vi "Extract Newtwork Variable.vi"(8 "Saving":bool[](array[boolean]), 9 "Current":dbl[](array[numeric]), 10 "Array in":i32[](array[numeric]), 11 "Array 3":T1[](array[typedef]) {"Unit Type" items=["", "Viper", "Hawk", "Other"]; "Current" format="%.2f"; "Day Cycle Count" format="%04d"}) -> (3 "Array out":T1[](array[typedef]) {"Unit Type" items=["", "Viper", "Hawk", "Other"]; "Current" format="%.2f"; "Day Cycle Count" format="%04d"})   [LabVIEW 2012]
uses:
  Nufi/Newfi LDN/Washer.ctl
  Nufi/Newfi LDN/Washer Details.ctl
  Nufi/Newfi LDN/Unit Type.ctl
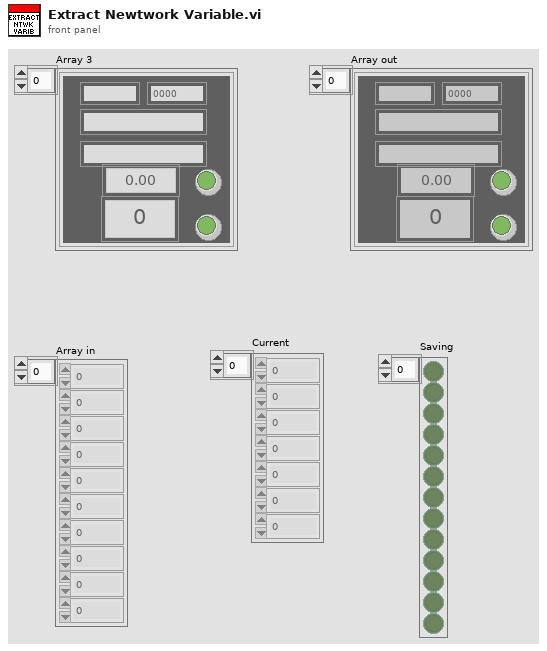
[diagram p1: front panel]
types:
  T1 = typedef "Washer.ctl" = cluster{"Serial Number":string, "Day Cycle Count":i32, "Station Label":string, "Status Color":u32, "Current Run Start Time":dbl, "Audit Alert":bool, "Washer Details":T2, "Board ID":string, "Boolean":bool, "RPM":u32, "Current":dbl, "Current Path":path, "Saving":bool, "Unit Type":T3}
  T2 = typedef "Washer Details.ctl" = cluster{"Cycle Count":string, "Status":string, "Notes":string, "Lab ID":string, "Total Time On":string, "TR Number":string}
  T3 = typedef "Unit Type.ctl" = u32
  T4 = cluster{"Serial Number":string, "Day Cycle Count":i32, "Station Label":string, "Status Color":u32, "Current Run Start Time":dbl, "Audit Alert":bool, "Washer Details":cluster{"Cycle Count":string, "Status":string, "Notes":string, "Lab ID":string, "Total Time On":string, "TR Number":string}, "Board ID":string, "Boolean":bool, "RPM":u32, "Current":dbl, "Current Path":path, "Saving":bool, "Unit Type":u32}
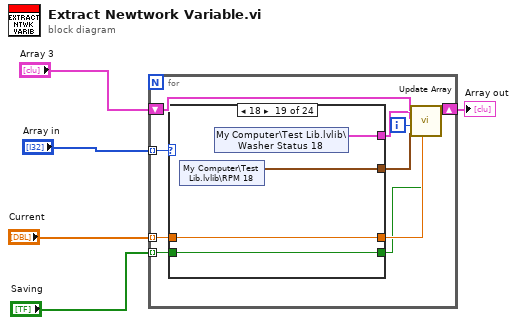
[diagram p0: block diagram]
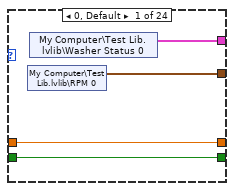
[diagram p2: hidden frame]
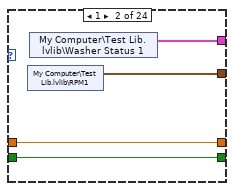
[diagram p3: hidden frame]
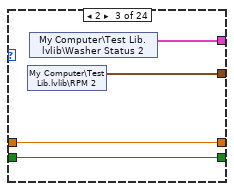
[diagram p4: hidden frame]
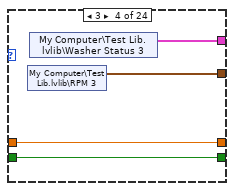
[diagram p5: hidden frame]
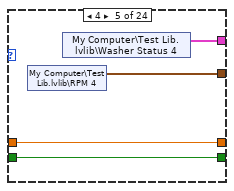
[diagram p6: hidden frame]
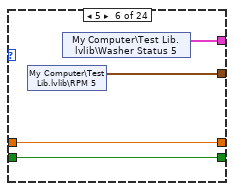
[diagram p7: hidden frame]
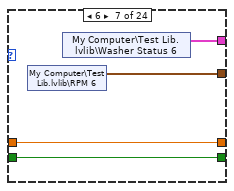
[diagram p8: hidden frame]
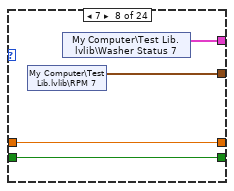
[diagram p9: hidden frame]
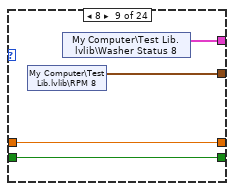
[diagram p10: hidden frame]
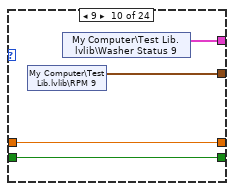
[diagram p11: hidden frame]
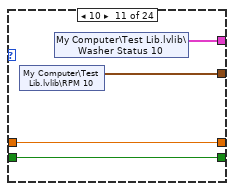
[diagram p12: hidden frame]
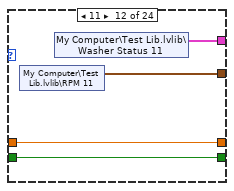
[diagram p13: hidden frame]
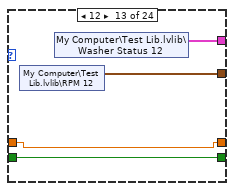
[diagram p14: hidden frame]
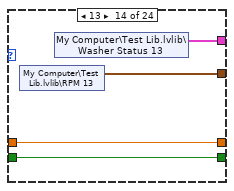
[diagram p15: hidden frame]
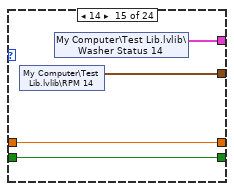
[diagram p16: hidden frame]
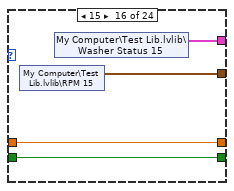
[diagram p17: hidden frame]
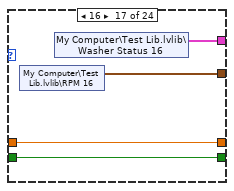
[diagram p18: hidden frame]
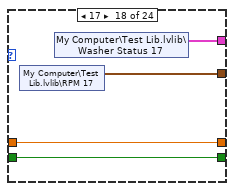
[diagram p19: hidden frame]
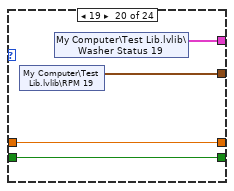
[diagram p20: hidden frame]
diagram:
  n1 = for {
    shift-right: [w14] -> w4
    shift-left: "Array 3" -> [w15]
    tunnel: "Array in" -> [w12] mode=indexing
    tunnel: "Current" -> [w9] mode=indexing
    tunnel: "Saving" -> [w7] mode=indexing
    i -> [w11]
    n2 = case shown="18" w12 {
      tunnel: [w19 w23 w27 w31 w35 w39 w43 w47 w51 w55 w59 w63 w67 w71 w75 w79 w83 w87 w91 w95 w99 w103 w107 w111] -> w13
      tunnel: [w18 w22 w26 w30 w34 w38 w42 w46 w50 w54 w58 w62 w66 w70 w74 w78 w82 w86 w90 w94 w98 w102 w106 w110] -> w10
      tunnel: [w17 w21 w25 w29 w33 w37 w41 w45 w49 w53 w57 w61 w65 w69 w73 w77 w81 w85 w89 w93 w97 w101 w105 w109] -> w8
      tunnel: w9 -> [w17 w21 w25 w29 w33 w37 w41 w45 w49 w53 w57 w61 w65 w69 w73 w77 w81 w85 w89 w93 w97 w101 w105 w109]
      tunnel: w7 -> [w16 w20 w24 w28 w32 w36 w40 w44 w48 w52 w56 w60 w64 w68 w72 w76 w80 w84 w88 w92 w96 w100 w104 w108]
      tunnel: [w16 w20 w24 w28 w32 w36 w40 w44 w48 w52 w56 w60 w64 w68 w72 w76 w80 w84 w88 w92 w96 w100 w104 w108] -> w6
      frame 0, Default {
        n3 = shared-variable "My Computer\\Test Lib.lvlib\\RPM 0"() -> (w18:cluster{"RPM":u32})  [unwired: 1 in, 1 out]
        n4 = shared-variable "My Computer\\Test Lib.lvlib\\Washer Status 0"() -> (w19:T4)  [unwired: 1 in, 1 out]
      }
      frame 1 {
        n5 = shared-variable "My Computer\\Test Lib.lvlib\\RPM1"() -> (w22:cluster{"RPM":u32})  [unwired: 1 in, 1 out]
        n6 = shared-variable "My Computer\\Test Lib.lvlib\\Washer Status 1"() -> (w23:T4)  [unwired: 1 in, 1 out]
      }
      frame 2 {
        n7 = shared-variable "My Computer\\Test Lib.lvlib\\RPM 2"() -> (w26:cluster{"RPM":u32})  [unwired: 1 in, 1 out]
        n8 = shared-variable "My Computer\\Test Lib.lvlib\\Washer Status 2"() -> (w27:T4)  [unwired: 1 in, 1 out]
      }
      frame 3 {
        n9 = shared-variable "My Computer\\Test Lib.lvlib\\RPM 3"() -> (w30:cluster{"RPM":u32})  [unwired: 1 in, 1 out]
        n10 = shared-variable "My Computer\\Test Lib.lvlib\\Washer Status 3"() -> (w31:T4)  [unwired: 1 in, 1 out]
      }
      frame 4 {
        n11 = shared-variable "My Computer\\Test Lib.lvlib\\RPM 4"() -> (w34:cluster{"RPM":u32})  [unwired: 1 in, 1 out]
        n12 = shared-variable "My Computer\\Test Lib.lvlib\\Washer Status 4"() -> (w35:T4)  [unwired: 1 in, 1 out]
      }
      frame 5 {
        n13 = shared-variable "My Computer\\Test Lib.lvlib\\RPM 5"() -> (w38:cluster{"RPM":u32})  [unwired: 1 in, 1 out]
        n14 = shared-variable "My Computer\\Test Lib.lvlib\\Washer Status 5"() -> (w39:T4)  [unwired: 1 in, 1 out]
      }
      frame 6 {
        n15 = shared-variable "My Computer\\Test Lib.lvlib\\RPM 6"() -> (w42:cluster{"RPM":u32})  [unwired: 1 in, 1 out]
        n16 = shared-variable "My Computer\\Test Lib.lvlib\\Washer Status 6"() -> (w43:T4)  [unwired: 1 in, 1 out]
      }
      frame 7 {
        n17 = shared-variable "My Computer\\Test Lib.lvlib\\RPM 7"() -> (w46:cluster{"RPM":u32})  [unwired: 1 in, 1 out]
        n18 = shared-variable "My Computer\\Test Lib.lvlib\\Washer Status 7"() -> (w47:T4)  [unwired: 1 in, 1 out]
      }
      frame 8 {
        n19 = shared-variable "My Computer\\Test Lib.lvlib\\RPM 8"() -> (w50:cluster{"RPM":u32})  [unwired: 1 in, 1 out]
        n20 = shared-variable "My Computer\\Test Lib.lvlib\\Washer Status 8"() -> (w51:T4)  [unwired: 1 in, 1 out]
      }
      frame 9 {
        n21 = shared-variable "My Computer\\Test Lib.lvlib\\RPM 9"() -> (w54:cluster{"RPM":u32})  [unwired: 1 in, 1 out]
        n22 = shared-variable "My Computer\\Test Lib.lvlib\\Washer Status 9"() -> (w55:T4)  [unwired: 1 in, 1 out]
      }
      frame 10 {
        n23 = shared-variable "My Computer\\Test Lib.lvlib\\RPM 10"() -> (w58:cluster{"RPM":u32})  [unwired: 1 in, 1 out]
        n24 = shared-variable "My Computer\\Test Lib.lvlib\\Washer Status 10"() -> (w59:T4)  [unwired: 1 in, 1 out]
      }
      frame 11 {
        n25 = shared-variable "My Computer\\Test Lib.lvlib\\RPM 11"() -> (w62:cluster{"RPM":u32})  [unwired: 1 in, 1 out]
        n26 = shared-variable "My Computer\\Test Lib.lvlib\\Washer Status 11"() -> (w63:T4)  [unwired: 1 in, 1 out]
      }
      frame 12 {
        n27 = shared-variable "My Computer\\Test Lib.lvlib\\RPM 12"() -> (w66:cluster{"RPM":u32})  [unwired: 1 in, 1 out]
        n28 = shared-variable "My Computer\\Test Lib.lvlib\\Washer Status 12"() -> (w67:T4)  [unwired: 1 in, 1 out]
      }
      frame 13 {
        n29 = shared-variable "My Computer\\Test Lib.lvlib\\RPM 13"() -> (w70:cluster{"RPM":u32})  [unwired: 1 in, 1 out]
        n30 = shared-variable "My Computer\\Test Lib.lvlib\\Washer Status 13"() -> (w71:T4)  [unwired: 1 in, 1 out]
      }
      frame 14 {
        n31 = shared-variable "My Computer\\Test Lib.lvlib\\RPM 14"() -> (w74:cluster{"RPM":u32})  [unwired: 1 in, 1 out]
        n32 = shared-variable "My Computer\\Test Lib.lvlib\\Washer Status 14"() -> (w75:T4)  [unwired: 1 in, 1 out]
      }
      frame 15 {
        n33 = shared-variable "My Computer\\Test Lib.lvlib\\RPM 15"() -> (w78:cluster{"RPM":u32})  [unwired: 1 in, 1 out]
        n34 = shared-variable "My Computer\\Test Lib.lvlib\\Washer Status 15"() -> (w79:T4)  [unwired: 1 in, 1 out]
      }
      frame 16 {
        n35 = shared-variable "My Computer\\Test Lib.lvlib\\RPM 16"() -> (w82:cluster{"RPM":u32})  [unwired: 1 in, 1 out]
        n36 = shared-variable "My Computer\\Test Lib.lvlib\\Washer Status 16"() -> (w83:T4)  [unwired: 1 in, 1 out]
      }
      frame 17 {
        n37 = shared-variable "My Computer\\Test Lib.lvlib\\RPM 17"() -> (w86:cluster{"RPM":u32})  [unwired: 1 in, 1 out]
        n38 = shared-variable "My Computer\\Test Lib.lvlib\\Washer Status 17"() -> (w87:T4)  [unwired: 1 in, 1 out]
      }
      frame 18 {
        n39 = shared-variable "My Computer\\Test Lib.lvlib\\RPM 18"() -> (w90:cluster{"RPM":u32})  [unwired: 1 in, 1 out]
        n40 = shared-variable "My Computer\\Test Lib.lvlib\\Washer Status 18"() -> (w91:T4)  [unwired: 1 in, 1 out]
      }
      frame 19 {
        n41 = shared-variable "My Computer\\Test Lib.lvlib\\RPM 19"() -> (w94:cluster{"RPM":u32})  [unwired: 1 in, 1 out]
        n42 = shared-variable "My Computer\\Test Lib.lvlib\\Washer Status 19"() -> (w95:T4)  [unwired: 1 in, 1 out]
      }
      frame 20 {
        n43 = shared-variable "My Computer\\Test Lib.lvlib\\RPM 20"() -> (w98:cluster{"RPM":u32})  [unwired: 1 in, 1 out]
        n44 = shared-variable "My Computer\\Test Lib.lvlib\\Washer Status 20"() -> (w99:T4)  [unwired: 1 in, 1 out]
      }
      frame 21 {
        n45 = shared-variable "My Computer\\Test Lib.lvlib\\RPM 21"() -> (w102:cluster{"RPM":u32})  [unwired: 1 in, 1 out]
        n46 = shared-variable "My Computer\\Test Lib.lvlib\\Washer Status 21"() -> (w103:T4)  [unwired: 1 in, 1 out]
      }
      frame 22 {
        n47 = shared-variable "My Computer\\Test Lib.lvlib\\RPM 22"() -> (w106:cluster{"RPM":u32})  [unwired: 1 in, 1 out]
        n48 = shared-variable "My Computer\\Test Lib.lvlib\\Washer Status 22"() -> (w107:T4)  [unwired: 1 in, 1 out]
      }
      frame 23 {
        n49 = shared-variable "My Computer\\Test Lib.lvlib\\RPM 23"() -> (w110:cluster{"RPM":u32})  [unwired: 1 in, 1 out]
        n50 = shared-variable "My Computer\\Test Lib.lvlib\\Washer Status 23"() -> (w111:T4)  [unwired: 1 in, 1 out]
      }
    }
    n51 = call "Update Array.vi"("Saving"=w6, "Current"=w8, "RPM and Station ID 0"=w10, "Row Index"=w11, "Washer Out"=w13, "Array IN"=w15) -> ("Array OUT"=w14:T1[])  [unwired: 5 in]
  }
  "Array out" <- w4
